vi "Test Customer Pick Up Order Broadcasts Status Update.vi"(8 "error in (no error)":errorcluster, 11 "Customer Test in":refnum<class "Customer Test.lvclass">) -> (0 "error out":errorcluster, 3 "Customer Test out":refnum<class "Customer Test.lvclass">)   [LabVIEW 2020, in "Customer Test.lvclass"]
uses:
  Customer Test.lvclass
  C:/Program Files (x86)/National Instruments/LabVIEW 2020/vi.lib/Asteme/LUnit/Test Case.lvclass
  Customer/Customer.lvclass
  C:/Program Files (x86)/National Instruments/LabVIEW 2020/vi.lib/Asteme/Triarc Framework/Process/Process.lvclass
  Support/Beverages/Beverage/Beverage.lvclass
  <vilib>/Asteme/Triarc Framework/Process/Process.lvclass/Process.ctl
  <vilib>/Asteme/LUnit/Test Case.lvclass/Test Case.ctl
  <vilib>/Asteme/LUnit/LUnit Assertion Result.lvclass/LUnit Assertion Result.ctl
  <vilib>/Asteme/Triarc Framework Test Suite/Support/Execution timer.vi
  <vilib>/Asteme/Triarc Framework/Process/Private/SubVIs/Wait for finish.vi
  <vilib>/Asteme/Triarc Framework/Process/Protected/Messaging/Enqueue Message.vi
  <vilib>/Asteme/Triarc Framework/Process/Private/SubVIs/Set Lifecycle State.vi
  <vilib>/Asteme/Triarc Framework/Process/Public/Lifecycle/Get Lifecycle State.vi
  <vilib>/Asteme/LUnit/Palette/Pass If.vi
  <vilib>/Asteme/LUnit/Set Assertion Type.vi
  <vilib>/AdvancedString/1D String Array to Delimited String.vi
  <vilib>/Asteme/LUnit/Palette/Fail.vi
  <vilib>/Asteme/LUnit/Palette/Pass.vi
  <vilib>/Asteme/LUnit/LUnit Write Assertion Type.vi
  <vilib>/Asteme/LUnit/Add test result.vi
  <vilib>/Asteme/LUnit/LUnit Write Passed.vi
  <vilib>/Asteme/LUnit/LUnit Get Test Case.vi
  <vilib>/Asteme/LUnit/Assertion Result/LUnit Get Test Name.vi
  <vilib>/Asteme/LUnit/LUnit Write Message.vi
  <vilib>/Asteme/LUnit/LUnit Write Description.vi
  <vilib>/Asteme/LUnit/Read Test Case Name.vi
  <vilib>/Asteme/Triarc Framework Test Suite/Support/Event Helpers/Dequeue Event Message.vi
  <vilib>/Utility/error.llb/Error Cluster From Error Code.vi
  <vilib>/Asteme/LUnit/LUnit Assertion Result.lvclass
  <vilib>/Asteme/Triarc Framework/Process/Process.lvclass
  <vilib>/Asteme/Triarc Framework Test Suite/Support/Event Helpers/Event Helpers.lvlib
  C:/Users/anton/Documents/GitHub/Triarc-Examples/Coffee Shop/Person/Person.lvclass
  C:/Program Files (x86)/National Instruments/LabVIEW 2020/vi.lib/Asteme/Triarc Framework/View/View.lvclass
  C:/Program Files (x86)/National Instruments/LabVIEW 2020/vi.lib/Asteme/Triarc Framework/Base/Base.lvclass
  C:/Program Files (x86)/National Instruments/LabVIEW 2020/vi.lib/Asteme/Triarc Framework/Error Handler Interface/Error Handler Interface.lvclass
  C:/Program Files (x86)/National Instruments/LabVIEW 2020/vi.lib/Asteme/Triarc Framework/Logging/Logging.lvclass
  C:/Users/anton/Documents/GitHub/Triarc-Examples/Coffee Shop/Customer/Customer.lvclass
  C:/Program Files (x86)/National Instruments/LabVIEW 2020/vi.lib/Asteme/Triarc Framework/Asynchronous Action/Async Action.lvclass
  C:/Users/anton/Documents/GitHub/Triarc-Examples/Coffee Shop/Process Job/Job Handler.lvclass
  <vilib>/Asteme/LUnit/Test Case.lvclass
  C:/Users/anton/Documents/GitHub/Triarc-Examples/Coffee Shop/Person Test/Person Test.lvclass
  C:/Program Files (x86)/National Instruments/LabVIEW 2020/vi.lib/Asteme/Triarc Framework Test Suite/View Test/View Test.lvclass
  C:/Program Files (x86)/National Instruments/LabVIEW 2020/vi.lib/Asteme/Triarc Framework Test Suite/Process Test/Process Test.lvclass
  C:/Program Files (x86)/National Instruments/LabVIEW 2020/vi.lib/Asteme/Triarc Framework Test Suite/Base Class Test/Base Test.lvclass
  C:/Users/anton/Documents/GitHub/Triarc-Examples/Coffee Shop/Customer Test/Customer Test.lvclass
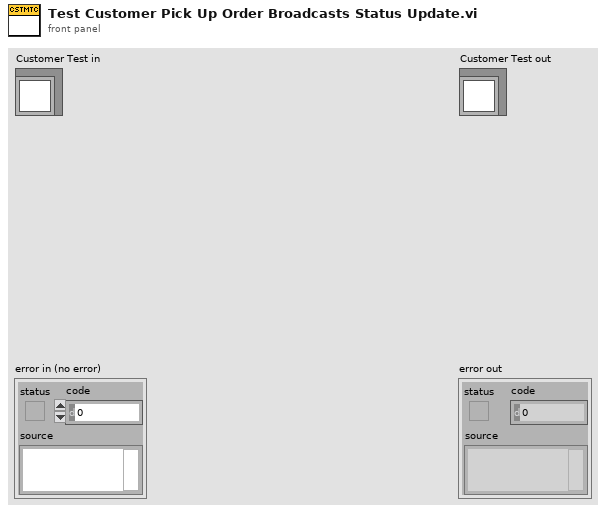
[diagram p1: front panel]
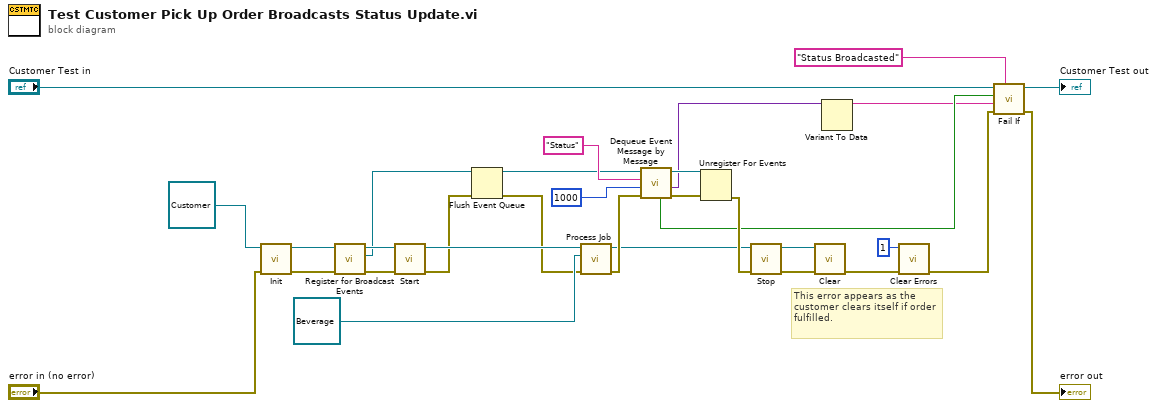
[diagram p0: block diagram]
diagram:
  # "This error appears as the customer clears itself if order fulfilled."
  n1 = call-dynamic "Init.vi"("error in (no error)"="error in (no error)", "View In"=refnum<class "Customer.lvclass"> refnum ("Customer.lvclass")) -> ("error out"=w28:errorcluster, "View Out"=w5:refnum<class "Customer.lvclass">)  [unwired: 8 in]
  n2 = call <vilib>:"Register for Broadcast Events.vi"("error in (no error)"=w28, "Process In"=w5) -> ("error out"=w30:errorcluster, "Event Registration Refnum Out"=w10:refnum<event-registration>, "Process Out"=w29:refnum<class "Customer.lvclass">)  [unwired: 7 in]
  n3 = call <vilib>:"Start.vi"("error in (no error)"=w30, "Process In"=w29) -> ("error out"=w24:errorcluster, "Process Out"=w25:refnum<class "Customer.lvclass">)  [unwired: 8 in]
  n4 = Flush Event Queue(0:w10, 3:w24) -> (8:w9:refnum<event-registration>, 11:w11:errorcluster)  [unwired: 4 in, 1 out]
  n5 = call-dynamic "Process Job.vi"("error in (no error)"=w11, "Task"=refnum<class "Beverage.lvclass"> refnum ("Beverage.lvclass"), "Work Dispatcher In"=w25) -> ("error out"=w23:errorcluster, "Work Dispatcher Out"=w3:refnum<class "Customer.lvclass">)  [unwired: 7 in]
  n6 = call <vilib>:"Dequeue Event Message by Message.vi"("error in (no error)"=w23, "Timeout (-1)"=1000, "Message"="Status", "Event Registration Refnum"=w9) -> ("error out"=w22:errorcluster, "Message Data"=w7:variant, "Event Registration Refnum Out"=w15:refnum<event-registration>, "Timed Out?"=w8:bool)  [unwired: 3 in, 1 out]
  n7 = Unregister For Events(event registration refnum=w15, error in=w22) -> (error out=w19:errorcluster)
  n8 = call <vilib>:"Stop.vi"("error in (no error)"=w19, "Process In"=w3) -> ("error out"=w27:errorcluster, "Process In"=w4:refnum<class "Customer.lvclass">)  [unwired: 7 in, 1 out]
  n9 = call-dynamic "Clear.vi"("error in (no error)"=w27, "View In"=w4) -> ("error out"=w18:errorcluster)  [unwired: 9 in]
  n10 = Variant To Data(Variant=w7) -> (data=w6:string)  [unwired: 2 in, 1 out]
  n11 = call <vilib>:"Clear Errors.vi"("error in (no error)"=w18, "specific error code to clear (0: all)"=1) -> ("error out"=w2:errorcluster)  [unwired: 4 in, 1 out]
  n12 = call <vilib>:"Fail If.vi"("Description"="Status Broadcasted", "error in (no error)"=w2, "Message"=w6, "Fail?"=w8, "Test Case In"="Customer Test in") -> ("error out"=→"error out":errorcluster, "Test Case Out"=→"Customer Test out":refnum<class "Customer Test.lvclass">)  [unwired: 5 in]
